vi "Stop Core.vi"(10 "final error code":i32, 11 "CS++ObjectManager in":refnum<class "CS++ObjectManager.lvclass">) -> (3 "CS++ObjectManager out":refnum<class "CS++ObjectManager.lvclass">)   [LabVIEW 2015, in "CS++ObjectManager.lvlib" / "CS++ObjectManager.lvclass"]
doc: "(<B>Filename</B>: Actor Framework.lvlib:Actor.lvclass:Stop Core.vi)\n\nDefines what the actor does before it stops. Use the <B>final error code</B> input to determine whether the actor shut down in response to an error.\n\nBy default, this method does nothing. A descendant class may override it to define behavior, such as shutting down any processes the actor initiated in its override of the Actor Core method."
uses:
  CS++ObjectManager.lvclass
  CS++ObjectManager.lvclass/CS++ObjectManager.ctl
  <vilib>/ActorFramework/Time-Delayed Send Message/Time-Delay Override Options.ctl
  CSPP_Core/Actors/CS++GUIActor/CS++GUIActor.lvclass
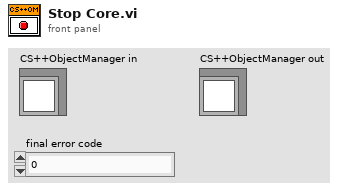
[diagram p1: front panel]
types:
  T1 = typedef "Time-Delay Override Options.ctl" = enum16{"Send next copy now", "Skip next scheduled copy", "Send next copy now and stop all further copies", "Stop all further copies"}
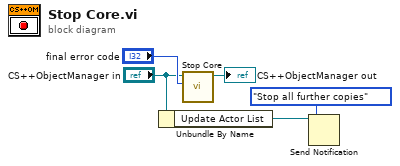
[diagram p0: block diagram]
diagram:
  n1 = Unbundle By Name("CS++ObjectManager in") -> ("Update Actor List"=w2:refnum<notifier>)
  n2 = call-parent "Stop Core.vi"("final error code"="final error code", "CS++GUIActor in"="CS++ObjectManager in") -> ("CS++GUIActor out"=→"CS++ObjectManager out":refnum<class "CS++ObjectManager.lvclass">)  [unwired: 9 in]
  n3 = Send Notification(notification=Time-Delay_Override_Options."Stop all further copies", notifier=w2) -> ()  [unwired: 1 in, 2 out]
